vi "Edge Detection_Highest Pixel Value.vi"   [LabVIEW 2016]
uses:
  <vilib>/vision/driver/NI_Vision_Acquisition_Software.lvlib
  <vilib>/userdefined/High Color/IMAQdx.ctl
  <vilib>/vision/NI_Vision_Development_Module.lvlib
types:
  T1 = typedef "IMAQdx.ctl" = refnum<k21>
  T2 = typedef "IMAQ Image.ctl" = refnum<image>
  T3 = typedef "ROI Descriptor" = cluster{"Global Rectangle":i32[], "Contours":cluster{"ID":enum32{"External", "Internal"}, "Type":u32, "Coordinates":i32[]}[]}
  T4 = typedef "Edge New.ctl" = cluster{"Location (Pixel)":cluster{"X":sgl, "Y":sgl}, "Location (Real-World)":cluster{"X":sgl, "Y":sgl}, "Distance (Pixel)":dbl, "Distance (Real-World)":dbl, "Strength":dbl, "Noise":dbl, "Rising?":bool}
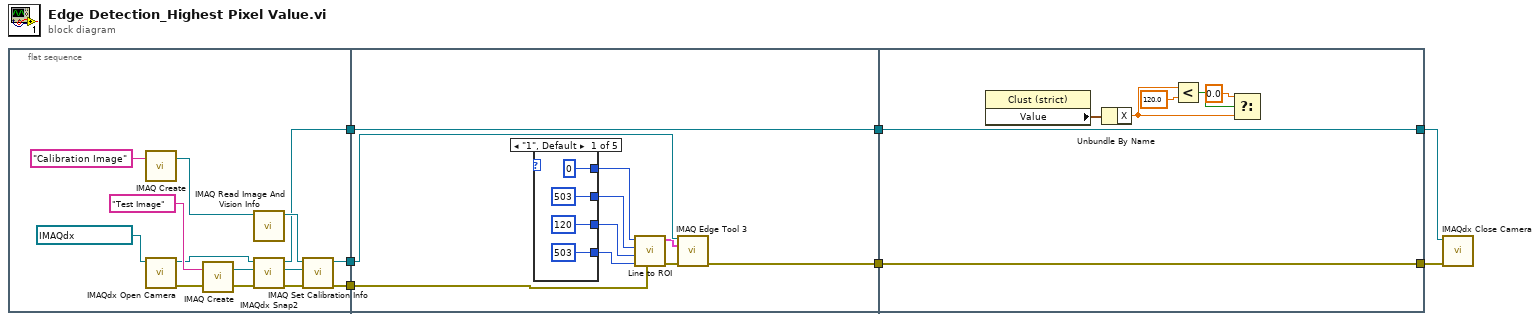
[diagram p0: block diagram]
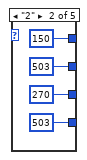
[diagram p2: hidden frame]
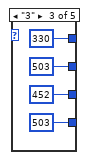
[diagram p3: hidden frame]
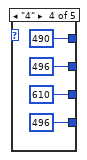
[diagram p4: hidden frame]
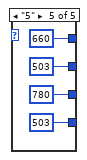
[diagram p5: hidden frame]
diagram:
  n1 = flat-sequence {
    tunnel: [w8] -> w7
    tunnel: [w10] -> w6
    tunnel: [w9] -> w5
    tunnel: w7 -> [w35]
    tunnel: w6 -> [w29]
    tunnel: w5 -> [w33]
    tunnel: [w35] -> w4
    tunnel: [w32] -> w3
    tunnel: [w63] -> w1
    tunnel: [w64] -> w2
    tunnel: w4 -> [w64]
    tunnel: w3 -> [w63]
    frame #0 {
      n2 = call "IMAQ Create"("Image Name"="Calibration Image") -> ("New Image"=w22:T2)  [unwired: 4 in, 1 out]
      n3 = call <vilib>:"IMAQdx Open Camera.vi"("Session In"=T1 "acA780-75gc") -> ("error out"=w16:errorcluster, "Session Out"=w12:T1, "error in"=w15:errorcluster)  [unwired: 8 in]
      n4 = call "IMAQ Create"("Image Name"="Test Image", "error in (no error)"=w16) -> ("New Image"=w13:T2, "error out"=w17:errorcluster)  [unwired: 3 in]
      n5 = call "IMAQ Read Image And Vision Info"("Image"=w22) -> ("Image Out"=w20:T2, "File Path"=w21:path)  [unwired: 7 in, 2 out]
      n6 = call <vilib>:"IMAQdx Snap2.vi"("error in"=w17, "Image In"=w13, "Session In"=w12) -> ("error out"=w18:errorcluster, "Image Out"=w19:T2, "Session Out"=w8:T1)  [unwired: 6 in]
      n7 = call "IMAQ Set Calibration Info"("error in (no error)"=w18, "Image Dst"=w19, "Image Src"=w20) -> ("error out"=w10:errorcluster, "Calibrated Image"=w9:T2)  [unwired: 7 in]
    }
    frame #1 {
      n8 = case shown="\"1\", Default" w34 {
        tunnel: [0 150 ("Start X") 330 ("Start X") 490 ("Start X") 660 ("Start X")] -> w27
        tunnel: [503 503 ("Start X") 503 ("Start X") 496 ("Start X") 503 ("Start X")] -> w26
        tunnel: [120 270 ("Start X") 452 ("Start X") 610 ("Start X") 780 ("Start X")] -> w25
        tunnel: [503 503 ("Start X") 503 ("Start X") 496 ("Start X") 503 ("Start X")] -> w24
        frame "1", Default {
        }
        frame "2" {
        }
        frame "3" {
        }
        frame "4" {
        }
        frame "5" {
        }
      }
      n9 = call "Line to ROI.vi"("error in (no error)"=w29, "End Y"=w24, "End X"=w25, "Start Y"=w26, "Start X"=w27) -> ("error out"=w28:errorcluster, "ROI Descriptor"=w30:T3)  [unwired: 5 in]
      n10 = call "IMAQ Edge Tool 3"("Image"=w33, "ROI Descriptor"=w30, "error in (no error)"=w28) -> ("Edge Information"=w31:T4[], "error out"=w32:errorcluster)  [unwired: 8 in, 3 out]
    }
    frame #2 {
      n11 = property class="Clust (strict)"() -> (reference=w56:refnum<vi>, "Value"=w57:cluster{"X":sgl, "Y":sgl})  [unwired: 1 in, 2 out]
      n12 = Unbundle By Name(w57) -> ("X"=w61:sgl)
      n13 = Less?(x=w61, y=sgl 120.0) -> (x < y?=w59:bool)
      n14 = Select(t=sgl 0.0, s=w59, f=w61) -> (s? t:f=w60:sgl)
    }
  }
  n15 = call <vilib>:"IMAQdx Close Camera.vi"("error in"=w1, "Session In"=w2) -> ()  [unwired: 9 in, 1 out]
